vi "test_launch-stopValidationWithMultipleTasks.vi"(11 "Test Case In":refnum<class "TaskControllerTests.lvclass">) -> (0 "error out":errorcluster, 3 "Test Case Out":refnum<class "TaskControllerTests.lvclass">)   [LabVIEW 2023, in "TaskControllerTests.lvclass"]
uses:
  TaskControllerTests.lvclass
  TaskControllerTests.lvclass/TaskControllerTests.ctl
  TaskMock/TaskMock.lvclass
  <vilib>/Astemes/LUnit/Test Case.lvclass
  source/TaskController/TaskController.lvclass
  C:/projects/TLC_Daemon/tests/TaskMock/TaskMock.lvclass
  C:/projects/TLC_Daemon/source/ITask/ITask.lvclass
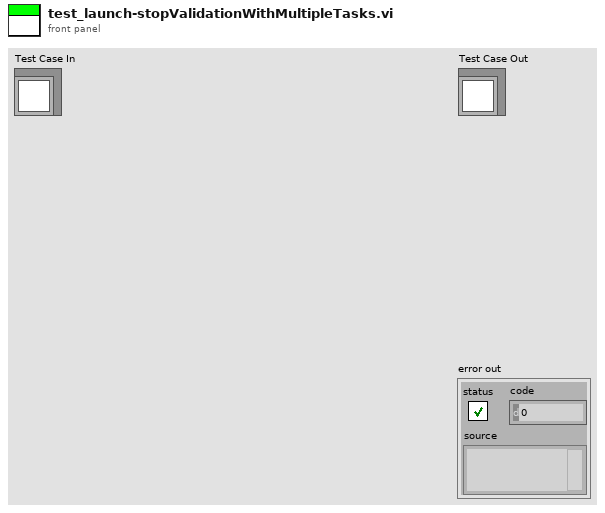
[diagram p1: front panel]
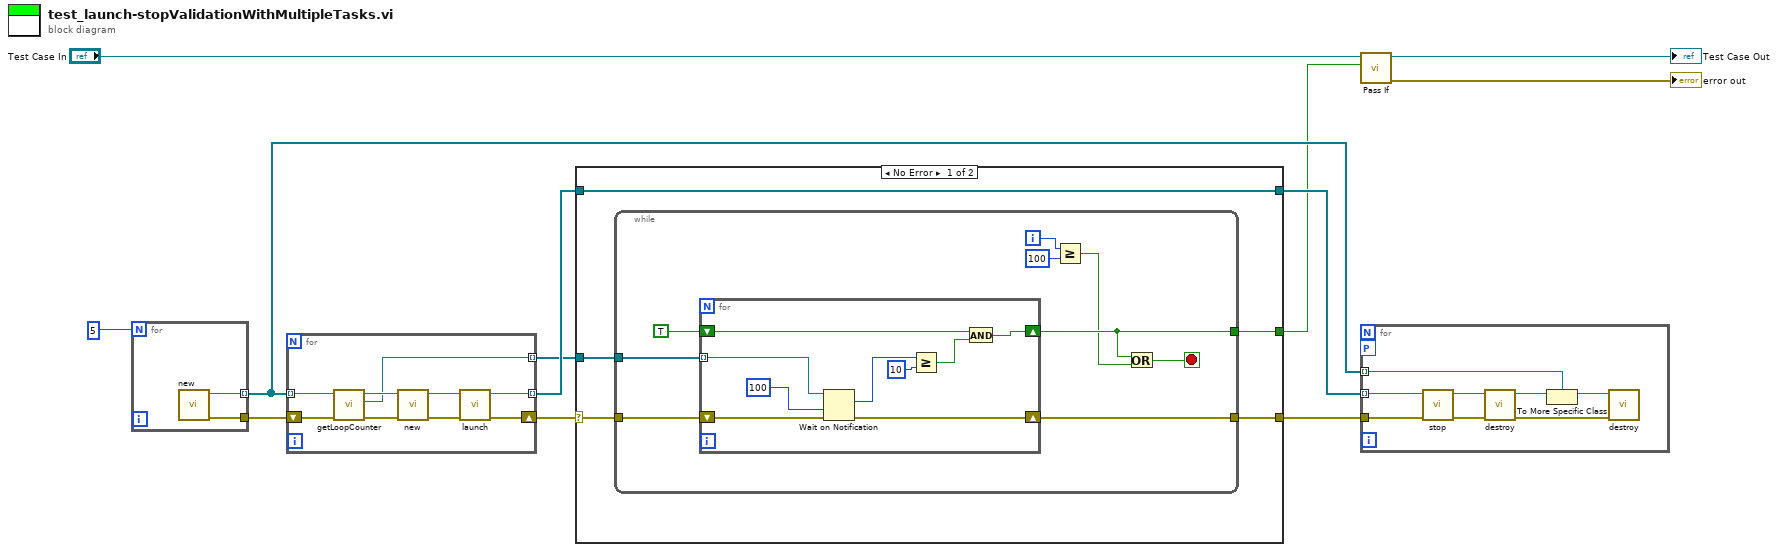
[diagram p0: block diagram]
diagram:
  n1 = for {
    N: 5 -> [_]
    tunnel: [w14] -> w4 mode=indexing
    tunnel: [w13] -> w2
    n2 = call "new.vi"() -> ("error out"=w13:errorcluster, "TaskMock out"=w14:refnum<class "TaskMock.lvclass">)  [unwired: 10 in]
  }
  n3 = for {
    tunnel: [w21] -> w9 mode=indexing
    tunnel: [w18] -> w7 mode=indexing
    tunnel: w4 -> [w17] mode=indexing
    shift-right: [w20] -> w8
    shift-left: w2 -> [w16]
    n4 = call "getLoopCounter.vi"("error in (no error)"=w16, "TaskMock in"=w17) -> ("error out"=w15:errorcluster, "loopCounter"=w18:refnum<notifier>, "TaskMock out"=w19:refnum<class "TaskMock.lvclass">)  [unwired: 7 in]
    n5 = call "new.vi"("error in (no error)"=w15, "task"=w19) -> ("error out"=w22:errorcluster, "TaskController out"=w23:refnum<class "TaskController.lvclass">)  [unwired: 8 in]
    n6 = call "launch.vi"("error in (no error)"=w22, "TaskController in"=w23) -> ("error out"=w20:errorcluster, "TaskController out"=w21:refnum<class "TaskController.lvclass">)  [unwired: 8 in]
  }
  n7 = case shown="No Error" w8 {
    selector: w8 -> [w28 _]
    tunnel: w9 -> [w26 w47]
    tunnel: w7 -> [w27 _]
    tunnel: [w26 w47] -> w6
    tunnel: [w25 _] -> w5
    tunnel: [w24 _] -> w3
    frame No Error {
      n8 = while {
        tunnel: w28 -> [w31]
        tunnel: w27 -> [w37]
        tunnel: [w34] -> w24
        tunnel: [w30] -> w25
        i -> [w36]
        stop <- w33 stop-if-true
        n9 = for {
          tunnel: w37 -> [w46] mode=indexing
          shift-right: [w40] -> w30
          shift-left: w31 -> [w41]
          shift-right: [w39] -> w34
          shift-left: TRUE -> [w38]
          n10 = Wait on Notification(notifier=w46, timeout in ms (-1)=100, error in (no error)=w41) -> (notification=w44:i32, error out=w40:errorcluster)  [unwired: 1 in, 2 out]
          n11 = Greater Or Equal?(x=w44, y=10) -> (x >= y?=w42:bool)
          n12 = And(x=w38, y=w42) -> (x .and. y?=w39:bool)
        }
        n13 = Greater Or Equal?(x=w36, y=100) -> (x >= y?=w32:bool)
        n14 = Or(x=w34, y=w32) -> (x .or. y?=w33:bool)
      }
    }
    frame Error {
    }
  }
  n15 = call <vilib>:"Pass If.vi"("Pass?"=w3, "LUnit Test Case In"="Test Case In") -> ("error out"=→"error out":errorcluster, "LUnit Test Case Out"=→"Test Case Out":refnum<class "TaskControllerTests.lvclass">)  [unwired: 8 in]
  n16 = for {
    tunnel: w6 -> [w55] mode=indexing
    tunnel: w5 -> [w54]
    tunnel: w4 -> [w51] mode=indexing
    workers-P: _ -> [_]
    n17 = call "stop.vi"("error in (no error)"=w54, "TaskController in"=w55) -> ("error out"=w52:errorcluster, "TaskController out"=w53:refnum<class "TaskController.lvclass">)  [unwired: 8 in]
    n18 = call "destroy.vi"("error in (no error)"=w52, "TaskController in"=w53) -> ("error out"=w50:errorcluster, "task"=w49:refnum<class "ITask.lvclass">)  [unwired: 8 in]
    n19 = To More Specific Class(target class=w51, reference=w49) -> (specific class reference=w48:refnum<class "TaskMock.lvclass">)  [unwired: 1 in, 1 out]
    n20 = call "destroy.vi"("error in (no error)"=w50, "TaskMock in"=w48) -> ()  [unwired: 9 in, 1 out]
  }
